vi "Fan Params.vi"(8 "error in":errorcluster, 10 "Fan Params Registers":map{string, u16}(c390), 11 "DeepU Results in":refnum<class "DeepU Results.lvclass">) -> (0 "error out":errorcluster, 3 "DeepU Results out":refnum<class "DeepU Results.lvclass">)   [LabVIEW 2019, in "Results.lvlib" / "DeepU Results.lvclass"]
uses:
  DeepU Results.lvclass
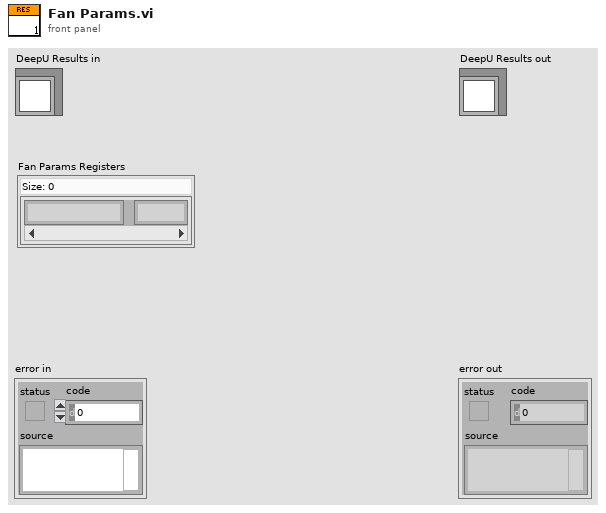
[diagram p1: front panel]
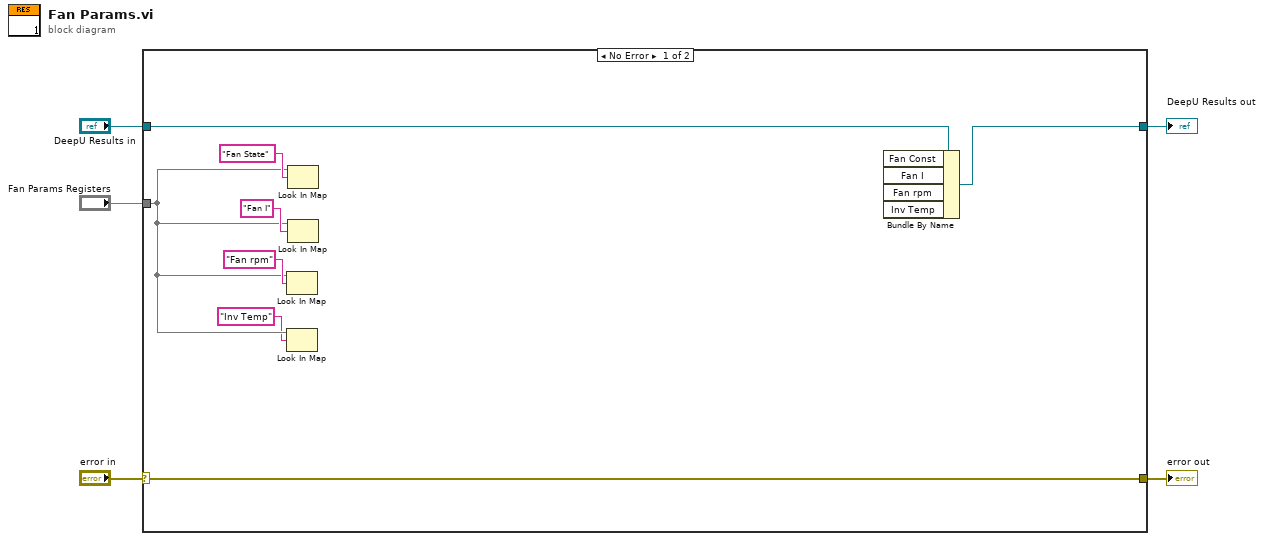
[diagram p0: block diagram]
diagram:
  n1 = case shown="No Error" "error in" {
    selector: "error in" -> [w12 w15]
    tunnel: [w12 w15] -> w4
    tunnel: [w11 w14] -> w2
    tunnel: "DeepU Results in" -> [w13 w14]
    tunnel: "Fan Params Registers" -> [w7 _]
    frame No Error {
      n2 = Look In Map(map=w7, key="Fan rpm") -> ()  [unwired: 1 in, 2 out]
      n3 = Look In Map(map=w7, key="Inv Temp") -> ()  [unwired: 1 in, 2 out]
      n4 = Look In Map(map=w7, key="Fan State") -> ()  [unwired: 1 in, 2 out]
      n5 = Look In Map(map=w7, key="Fan I") -> ()  [unwired: 1 in, 2 out]
      n6 = Bundle By Name(cluster=w13) -> (w11:refnum<class "DeepU Results.lvclass">)  [unwired: 4 in]
    }
    frame Error {
    }
  }
  "error out" <- w4
  "DeepU Results out" <- w2
